vi "Reorganize&ScaleMeasurements.vi"(6 "Meas Aperature":dbl=0.1 format="%#_13g", 8 "Error In":errorcluster, 9 "MeasurementType":string, 10 "SNMPDataAsStrings":string[](array[string])) -> (0 "Error Out":errorcluster, 1 "Numerical Information":bool, 2 "String Data":string, 3 "output waveform":waveform(dbl), 4 "Alarmed":bool)   [LabVIEW 2018, in "SensorPlugins.lvlib" / "RoomAlert.lvclass"]
doc: "This VI takes the raw measurements from the RoomAlert instrument, scales the measurements accordingly, and separates the measurements between numerical and string values."
uses:
  RoomAlert.lvclass
panel:
  out "Replaced":bool
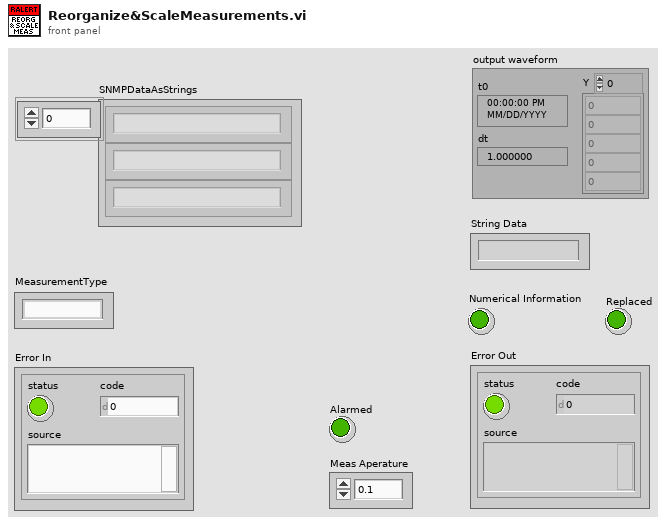
[diagram p1: front panel]
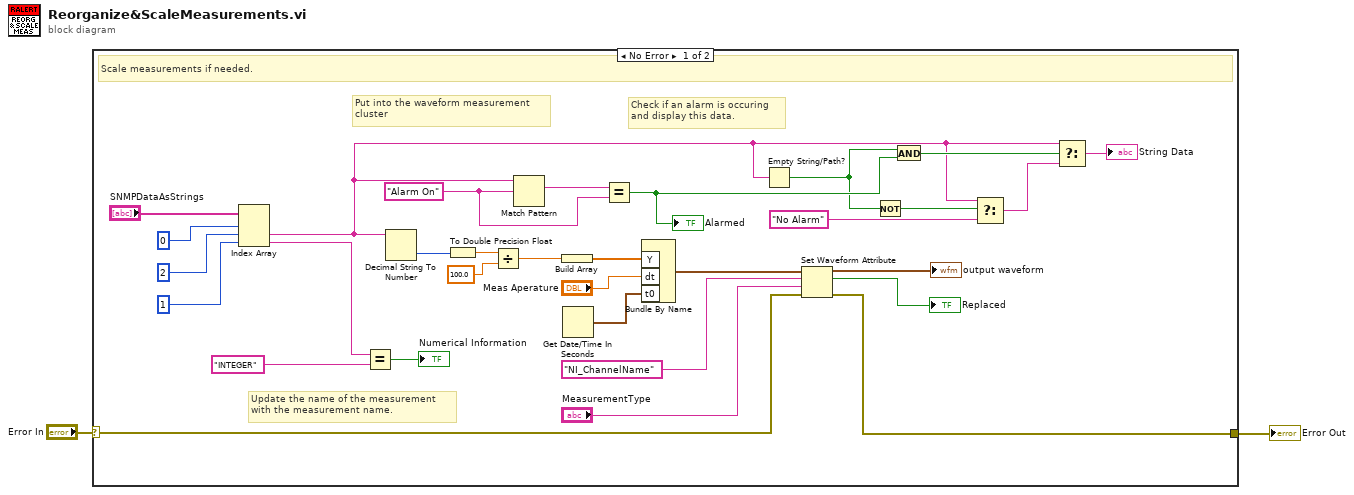
[diagram p0: block diagram]
diagram:
  n1 = case shown="No Error" "Error In" {
    selector: "Error In" -> [w9 w34]
    tunnel: [w29 w34] -> w2
    frame No Error {
      w14 = "Alarm On" ("regular expression")
      # "Check if an alarm is occuring\nand display this data."
      # "Update the name of the measurement \nwith the measurement name."
      # "Put into the waveform measurement\ncluster"
      # "Scale measurements if needed."
      n2 = Index Array(array="SNMPDataAsStrings", index #1=0 ("index"), index #2=2 ("disabled index (col)"), index #3=1 ("index (col)")) -> (element #2=w7:string, element #3=w16:string)  [unwired: 1 out]
      n3 = Equal?(x=w16, y="INTEGER" ("String")) -> (x = y?=→"Numerical Information":bool)
      n4 = Decimal String To Number(string=w7) -> (number=w20:i32)  [unwired: 2 in, 1 out]
      n5 = To Double Precision Float(number=w20) -> (double precision float=w19:dbl)
      n6 = Divide(x=w19, y=100.0 ("SNMPDataAsStrings")) -> (x/y=w10:dbl)
      n7 = Match Pattern(string=w7, regular expression=w14) -> (match substring=w15:string)  [unwired: 1 in, 3 out]
      n8 = Build Array(w10) -> (w21:dbl[])
      n9 = Get Date/Time In Seconds() -> (seconds since 1Jan1904=w33:timestamp)
      n10 = Equal?(x=w15, y=w14) -> (x = y?=w5:bool)
      "Alarmed" <- w5
      n11 = Bundle By Name("Y"=w21, "dt"="Meas Aperature", "t0"=w33) -> (w31:waveform(dbl))  [unwired: 1 in]
      n12 = Empty String/Path?(string/path=w7) -> (empty?=w4:bool)
      n13 = Set Waveform Attribute(4:w9, 5:"MeasurementType", 6:"NI_ChannelName" ("name"), 7:w31) -> (0:w29:errorcluster, 2:→"Replaced":bool, 3:→"output waveform":waveform(dbl))
      n14 = Not(x=w4) -> (.not. x?=w3:bool)
      n15 = And(x=w4, y=w5) -> (x .and. y?=w11:bool)
      n16 = Select(t=w7, s=w3, f="No Alarm" ("String Data")) -> (s? t:f=w6:string)
      n17 = Select(t=w7, s=w11, f=w6) -> (s? t:f=→"String Data":string)
    }
    frame Error {
    }
  }
  "Error Out" <- w2
